vi "SampleSensorLoop.vi"   [LabVIEW 2016]
uses:
  DisplacementData.ctl
  DisplacementStates.ctl
  DisplacementSample.ctl
  DisplacementErrorSample.ctl
  DisplacementErrorCodes.ctl
  <vilib>/Platform/TimedLoop/XDataNode/timing_clust.ctl
  <vilib>/Platform/TimedLoop/XDataNode/nitl_modes.ctl
  <vilib>/Platform/TimedLoop/XDataNode/wakeup.ctl
  <vilib>/rvi/Emulation/niFpgaSctlEmulationGetInTimedLoop.vi
  <vilib>/rvi/Emulation/niFpgaEmulationReportErrorSimple.vi
  <vilib>/rvi/Emulation/niFpgaGetClockAttributes.vi
  <vilib>/rvi/Emulation/niFpgaCriticalErrorInLSC.vi
  <vilib>/rvi/Emulation/niFpgaEmulationIsFPGAContextNoSignature.vi
  <vilib>/rvi/errors/niFpgaSetErrorForExecOnDevCompSimple.vi
  <vilib>/rvi/eio/common/nirviEmuReportErrorAndStop.vi
  <vilib>/rvi/DataTransferAndStorage/Container/Common/niFpgaContainerGetUniqueNameForEmu.vi
  <vilib>/rvi/FIFO/Fifo_Resource/nirvififoEmulationSetSize.vi
  <vilib>/rvi/FIFO/Fifo_Resource/nirviFifoEmulationQueueMgr.vi
  <instcachedir>/0/nirviFifoEmulationQueueMgr_E5CAEC123FF24DC58D834DCA3CDAA9B5.lvgen/nirviFifoEmulationQueueMgr_E5CAEC123FF24DC58D834DCA3CDAA9B5_004.vi
  <vilib>/Utility/error.llb/Clear Errors.vi
  <vilib>/rvi/FIFO/Fifo_Resource/nirvififoEmulationCreateLock.vi
  <vilib>/rvi/Emulation/niFpgaProcessEmulError.vi
  <vilib>/rvi/FIFO/Fifo_Resource/nirvififoEmulationObtainLock.vi
  <vilib>/rvi/FIFO/Fifo_Resource/nirvififoEmulationReleaseLock.vi
  <vilib>/rvi/occurrence/nirviWaitOnOccurrenceBase.vi
  <vilib>/rvi/errors/nirviReportUnexpectedCaseInternalError.vi
  <vilib>/rvi/errors/nirviReportUnexpectedCaseInternalError (U32).vi
  <vilib>/rvi/FIFO/Fifo_Resource/nirvififoEmulationDetermineInputValidOut.vi
  <instcachedir>/0/nirviFifoEmulationQueueMgr_E5CAEC123FF24DC58D834DCA3CDAA9B5.lvgen/nirviFifoEmulationQueueMgr_E5CAEC123FF24DC58D834DCA3CDAA9B5_009.vi
  <vilib>/rvi/Memory/Memory_Emulation/niFpgaMemoryEmulationCacheClearOnFirstRun.vi
  <vilib>/rvi/Memory/Memory_Emulation/nirvimemoryEmulationManagerCache_MakeExclusive.vi
  <vilib>/rvi/Memory/Memory_Emulation/niFpgaMemoryEmulationValidateCache.vi
  <vilib>/rvi/Memory/Memory_Emulation/nirvimemoryEmulationManagerCache_InsertValue.vi
  <vilib>/rvi/Memory/Memory_Emulation/nirvimemoryEmulationManagerCache_ReleaseExclusive.vi
  <vilib>/rvi/Memory/Memory_Emulation/nirvimemoryEmulationManagerCache_GetValue.vi
  <vilib>/rvi/Memory/Memory_Emulation/nirvimemoryEmulationManagerCache_SetValue.vi
  <vilib>/rvi/eio/common/nirviEmuTemplateMethod_errors.vi
  <instcachedir>/0/nirviFifoEmulationQueueMgr_E5CAEC123FF24DC58D834DCA3CDAA9B5.lvgen/nirviFifoEmulationQueueMgr_E5CAEC123FF24DC58D834DCA3CDAA9B5_028.vi
  <instcachedir>/0/nirviFifoEmulationQueueMgr_E5CAEC123FF24DC58D834DCA3CDAA9B5.lvgen/nirviFifoEmulationQueueMgr_E5CAEC123FF24DC58D834DCA3CDAA9B5_029.vi
  <vilib>/Platform/TimedLoop/XDataNode/XDataNode.xnode
  <vilib>/rvi/DataTransferAndStorage/Container/XNode/niFpgaContainer.xnode
  <vilib>/rvi/FIFO/Fifo_Resource/nirvififoEmulationRead.vi
  <vilib>/rvi/FIFO/Fifo_Resource/nirvififoEmulationWrite.vi
  <vilib>/rvi/DataTransferAndStorage/Register/Emulation/niFpgaRegisterEmulation.vi
  <vilib>/eio/EIONode/EIONode.xnode
  <vilib>/Platform/TimedLoop/XDataNode/XDNodeRunTimeDep.lvlib
types:
  T1 = typedef "DisplacementData.ctl" = cluster{"State":T2, "Sensor":u8, "Negative":bool, "Timestamp":u64, "ErrorNumber":u8, "Timeout":i32, "Sample":T3, "ErrorSample":T4}
  T2 = typedef "DisplacementStates.ctl" = enum16{"WaitForTrigger", "ClearRxFIFO", "WaitForClearComplete", "WriteM", "Write0", "WriteCR", "WriteNL", "ReadFirstCharacter", "ReadDataResponse", "ReadDeliminator", "ReadSign", "ReadHundreds", "ReadTens", "ReadOnes", "ReadDecimal", "ReadTenths", "ReadHundredths", "ReadThousandths", "ReadTenThousandths", "PrepareSample", "MoveSample", "ReadErrorR", "ReadErrorDeliminator1", "ReadErrorM", "ReadError0", "ReadErrorDeliminator2", "ReadErrorNumberTens", "ReadErrorNumberOnes", "ReadErrorCR", "ParseErrorNumber", "ResponseUnknownError", "ResponseInvalidError", "ResponseTimeoutError", "SensorIndicatesInvalidCommandError", "SensorIndicatesCommunicationTimeoutError", "SensorIndicatesDataLengthError", "SensorIndicatesNumberOfParametersError", "SensorIndicatesParameterError", "SensorIndicatesCommunicationError", "SensorIndicatesIDNumberError", "SensorIndicatesExpansionLineError", "SensorIndicatesWriteControlError", "PrepareErrorCode", "MoveErrorCode"}
  T3 = typedef "DisplacementSample.ctl" = cluster{"Timestamp":u64, "TxBytes":u64, "RxBytes":u64, "TxFrames":u64, "RxFrames":u64, "Sensor1Raw":i32, "Sensor2Raw":i32, "Sensor3Raw":i32, "Sensor4Raw":i32, "Sensor5Raw":i32, "Sensor6Raw":i32, "Sensor7Raw":i32, "Sensor8Raw":i32, "Sensor1Eng":sgl, "Sensor2Eng":sgl, "Sensor3Eng":sgl, "Sensor4Eng":sgl, "Sensor5Eng":sgl, "Sensor6Eng":sgl, "Sensor7Eng":sgl, "Sensor8Eng":sgl, "PositionX":sgl, "PositionY":sgl, "PositionZ":sgl, "RotationX":sgl, "RotationY":sgl, "RotationZ":sgl}
  T4 = typedef "DisplacementErrorSample.ctl" = cluster{"Timestamp":u64, "TxBytes":u64, "RxBytes":u64, "TxFrames":u64, "RxFrames":u64, "ErrorCode":T5}
  T5 = typedef "DisplacementErrorCodes.ctl" = enum16{"None", "ResponseUnknownError", "ResponseInvalidError", "ResponseTimeoutError", "SensorIndicatesInvalidCommandError", "SensorIndicatesCommunicationTimeoutError", "SensorIndicatesDataLengthError", "SensorIndicatesNumberOfParametersError", "SensorIndicatesParameterError", "SensorIndicatesCommunicationError", "SensorIndicatesIDNumberError", "SensorIndicatesExpansionLineError", "SensorIndicatesWriteControlError"}
  T6 = typedef "XDNodeRunTimeDep.lvlib/timing_clust.ctl" = cluster{"Expected End [f-1]":u64, "Actual End [f-1]":u64, "Finished Late? [f-1]":bool, "Expected End [i-1]":u64, "Actual End [i-1]":u64, "Finished Late? [i-1]":bool, "Expected Start [i]":u64, "Actual Start [i]":u64, "Expected Start [f]":u64, "Actual Start [f]":u64, "Source Name":string, "Structure Name":string, "Period":i64, "Deadline":i64, "Offset":i64, "Start":i64, "Priority":i32, "Timeout":i32, "Mode":T7, "Wakeup Reason":T8, "Error":errorcluster, "Source Type":string, "Secondary Source Type":string, "Global End Time":u64, "Global Start Time":u64, "Frame Duration":u64, "Iteration Duration":u64, "Assigned CPU":i32, "I/O Scan Engine Mode":u32}
  T7 = typedef "XDNodeRunTimeDep.lvlib/nitl_modes.ctl" = enum32{"No Change", "Process missed periods, maintain original phase", "Discard missed periods, maintain original phase", "Process missed periods, ignore original phase", "Discard missed periods, ignore original phase"}
  T8 = typedef "XDNodeRunTimeDep.lvlib/wakeup.ctl" = enum32{"Normal", "Aborted", "Asynchronous wakeup", "Timing source error", "Timed loop error", "Timeout"}
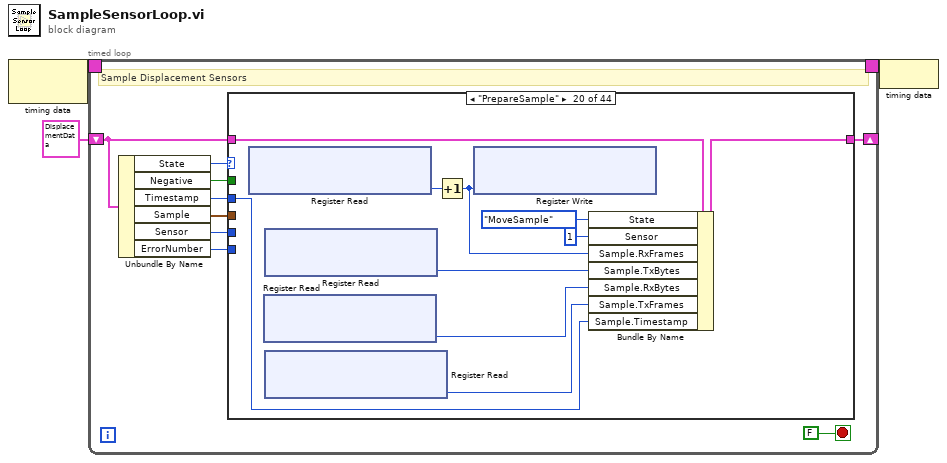
[diagram p0: block diagram]
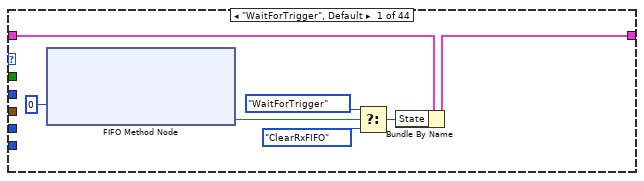
[diagram p2: hidden frame]
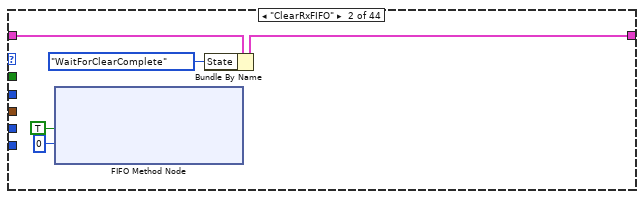
[diagram p3: hidden frame]
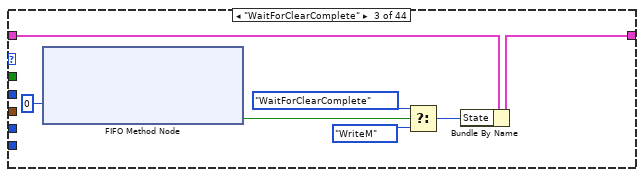
[diagram p4: hidden frame]
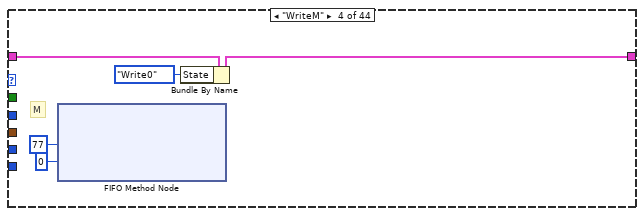
[diagram p5: hidden frame]
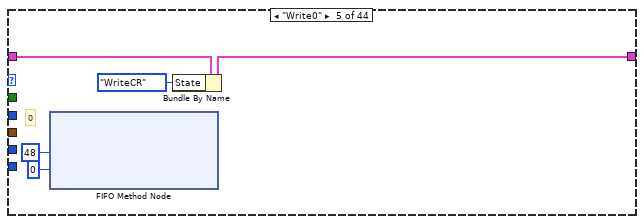
[diagram p6: hidden frame]
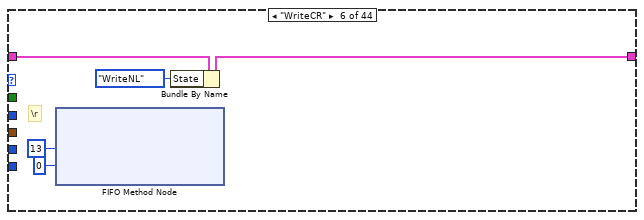
[diagram p7: hidden frame]
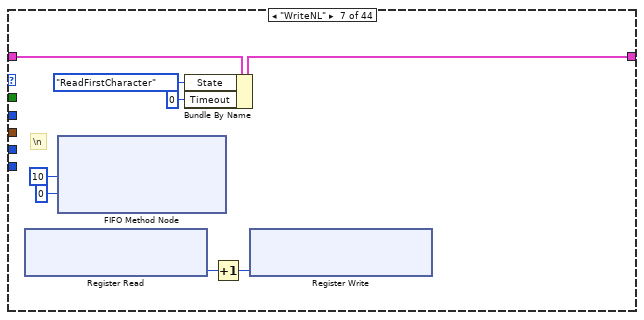
[diagram p8: hidden frame]
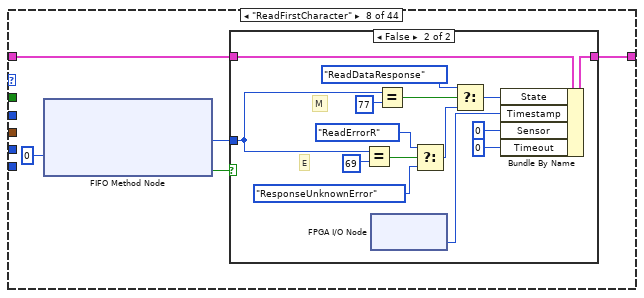
[diagram p9: hidden frame]
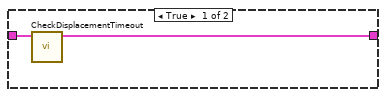
[diagram p10: hidden frame]
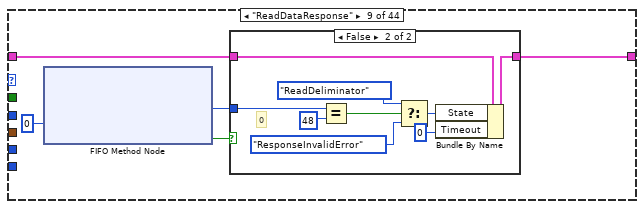
[diagram p11: hidden frame]
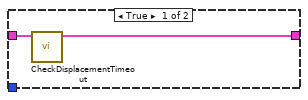
[diagram p12: hidden frame]
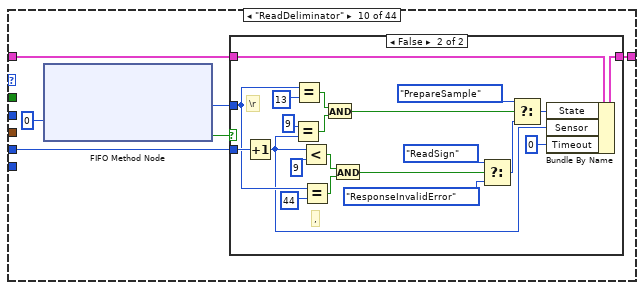
[diagram p13: hidden frame]
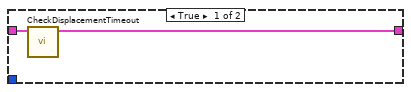
[diagram p14: hidden frame]
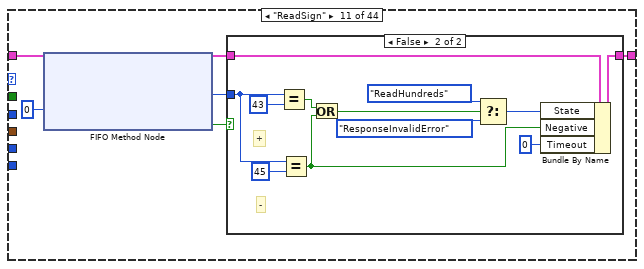
[diagram p15: hidden frame]
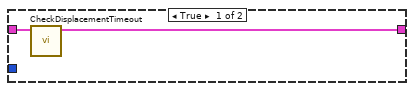
[diagram p16: hidden frame]
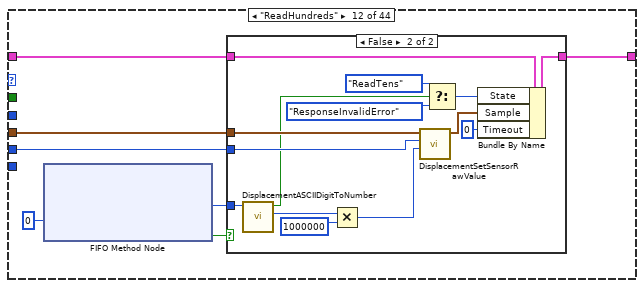
[diagram p17: hidden frame]
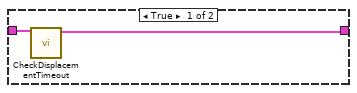
[diagram p18: hidden frame]
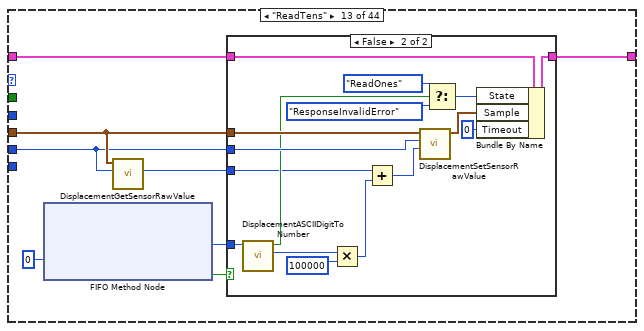
[diagram p19: hidden frame]
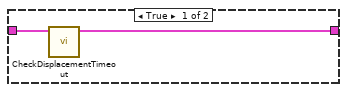
[diagram p20: hidden frame]
diagram:
  n1 = node-c288() -> (w3:T6)  [unwired: 1 in]
  n2 = timed-loop {
    timing: w3 -> [_]
    timing-out: [_] -> w2
    shift-right: [w12] -> _
    shift-left: T1 {"State"=enum."WaitForTrigger", "Sensor"=0, "Negative"=FALSE, "Timestamp"=0, "ErrorNumber"=0, "Timeout"=0, "Sample"={"Timestamp"=0, "TxBytes"=0, "RxBytes"=0, "TxFrames"=0, "RxFrames"=0, "Sensor1Raw"=0, "Sensor2Raw"=0, "Sensor3Raw"=0, "Sensor4Raw"=0, "Sensor5Raw"=0, "Sensor6Raw"=0, "Sensor7Raw"=0, "Sensor8Raw"=0, "Sensor1Eng"=0.0, "Sensor2Eng"=0.0, "Sensor3Eng"=0.0, "Sensor4Eng"=0.0, "Sensor5Eng"=0.0, "Sensor6Eng"=0.0, "Sensor7Eng"=0.0, "Sensor8Eng"=0.0, "PositionX"=0.0, "PositionY"=0.0, "PositionZ"=0.0, "RotationX"=0.0, "RotationY"=0.0, "RotationZ"=0.0}, "ErrorSample"={"Timestamp"=0, "TxBytes"=0, "RxBytes"=0, "TxFrames"=0, "RxFrames"=0, "ErrorCode"=enum."None"}} ("DisplacementData") -> [w11]
    stop <- FALSE stop-if-true
    # "Sample Displacement Sensors"
    n3 = Unbundle By Name(w11) -> ("State"=w10:T2, "Negative"=w9:bool, "Timestamp"=w7:u64, "Sample"=w8:T3, "Sensor"=w6:u8, "ErrorNumber"=w5:u8)
    n4 = case shown="\"PrepareSample\"" w10 {
      tunnel: [w16 w23 w30 w35 w40 w45 w53 w58 w80 w97 w125 w146 w170 w196 w219 w238 w264 w290 w316 w342 w349 w353 w369 w385 w401 w417 w433 w453 w472 w487 w501 w505 w509 w513 w517 w521 w525 w529 w533 w537 w541 w545 w555 w562] -> w12
      tunnel: w11 -> [w19 w24 w31 w36 w41 w46 w54 w59 w81 w98 w126 w147 w171 w197 w220 w239 w265 w291 w317 w343 w346 w354 w370 w386 w402 w418 w434 w454 w473 w488 w502 w506 w510 w514 w518 w522 w526 w530 w534 w538 w542 w546 w556 w559]
      tunnel: w9 -> [_ _ _ _ _ _ _ _ _ _ _ _ _ _ _ _ _ _ _ _ _ _ _ _ _ _ _ _ _ _ _ _ _ _ _ _ _ _ _ _ _ _ _ _]
      tunnel: w8 -> [_ _ _ _ _ _ _ _ _ _ _ w142 w166 w192 _ w234 w260 w286 w312 _ _ _ _ _ _ _ _ _ _ _ _ _ _ _ _ _ _ _ _ _ _ _ _ _]
      tunnel: w7 -> [_ _ _ _ _ _ _ _ _ _ _ _ _ _ _ _ _ _ _ w334 _ _ _ _ _ _ _ _ _ _ _ _ _ _ _ _ _ _ _ _ _ _ w547 _]
      tunnel: w6 -> [_ _ _ _ _ _ _ _ _ w93 _ w141 w165 w191 _ w233 w259 w285 w311 _ _ _ _ _ _ _ _ _ _ _ _ _ _ _ _ _ _ _ _ _ _ _ _ _]
      tunnel: w5 -> [_ _ _ _ _ _ _ _ _ _ _ _ _ _ _ _ _ _ _ _ _ _ _ _ _ _ _ w449 _ w485 _ _ _ _ _ _ _ _ _ _ _ _ _ _]
      frame "WaitForTrigger", Default {
        n5 = xnode ("FIFO Method Node")("Timeout"=0) -> ("Timed Out?"=w14:bool)  [unwired: 1 in, 2 out]
        n6 = Select(t=DisplacementStates."WaitForTrigger" ("DisplacementStates"), s=w14, f=DisplacementStates."ClearRxFIFO") -> (s? t:f=w17:T2)
        n7 = Bundle By Name(cluster=w19, "State"=w17) -> (w16:T1)
      }
      frame "ClearRxFIFO" {
        n8 = xnode ("FIFO Method Node")("Element"=TRUE, "Timeout"=0) -> ()  [unwired: 1 in, 2 out]
        n9 = Bundle By Name(cluster=w24, "State"=DisplacementStates."WaitForClearComplete") -> (w23:T1)
      }
      frame "WaitForClearComplete" {
        n10 = xnode ("FIFO Method Node")("Timeout"=0) -> ("Timed Out?"=w26:bool)  [unwired: 1 in, 2 out]
        n11 = Select(t=DisplacementStates."WaitForClearComplete" ("State"), s=w26, f=DisplacementStates."WriteM") -> (s? t:f=w28:T2)
        n12 = Bundle By Name(cluster=w31, "State"=w28) -> (w30:T1)
      }
      frame "WriteM" {
        # "M"
        n13 = xnode ("FIFO Method Node")("Element"=u8 77, "Timeout"=0) -> ()  [unwired: 1 in, 2 out]
        n14 = Bundle By Name(cluster=w36, "State"=DisplacementStates."Write0" ("f")) -> (w35:T1)
      }
      frame "Write0" {
        # "0"
        n15 = xnode ("FIFO Method Node")("Element"=u8 48, "Timeout"=0) -> ()  [unwired: 1 in, 2 out]
        n16 = Bundle By Name(cluster=w41, "State"=DisplacementStates."WriteCR" ("f")) -> (w40:T1)
      }
      frame "WriteCR" {
        # "\\r"
        n17 = xnode ("FIFO Method Node")("Element"=u8 13, "Timeout"=0) -> ()  [unwired: 1 in, 2 out]
        n18 = Bundle By Name(cluster=w46, "State"=DisplacementStates."WriteNL" ("f")) -> (w45:T1)
      }
      frame "WriteNL" {
        # "\\n"
        n19 = xnode ("Register Read")() -> ("Data"=w48:u64)  [unwired: 1 in, 1 out]
        n20 = xnode ("FIFO Method Node")("Element"=u8 10, "Timeout"=0) -> ()  [unwired: 1 in, 2 out]
        n21 = Bundle By Name(cluster=w54, "State"=DisplacementStates."ReadFirstCharacter", "Timeout"=0) -> (w53:T1)
        n22 = Increment(x=w48) -> (x+1=w49:u64)
        n23 = xnode ("Register Write")("Data"=w49) -> ()  [unwired: 1 in, 1 out]
      }
      frame "ReadFirstCharacter" {
        n24 = xnode ("FIFO Method Node")("Timeout"=0) -> ("Element"=w55:u8, "Timed Out?"=w56:bool)  [unwired: 1 in, 1 out]
        n25 = case shown="False" w56 {
          tunnel: w59 -> [w61 w76]
          tunnel: [w60 w75] -> w58
          tunnel: w55 -> [_ w68]
          frame True {
            n26 = call "CheckDisplacementTimeout.vi"("DisplacementData in"=w61) -> ("DisplacementData out"=w60:T1)  [unwired: 10 in]
          }
          frame False {
            # "E"
            # "M"
            n27 = Equal?(x=w68, y=u8 69) -> (x = y?=w69:bool)
            n28 = xnode "FPGA I/O Node"() -> ("Time"=w64:u64)  [unwired: 1 in, 1 out]
            n29 = Equal?(x=w68, y=u8 77) -> (x = y?=w73:bool)
            n30 = Select(t=DisplacementStates."ReadErrorR", s=w69, f=DisplacementStates."ResponseUnknownError") -> (s? t:f=w66:T2)
            n31 = Select(t=DisplacementStates."ReadDataResponse" ("State"), s=w73, f=w66) -> (s? t:f=w72:T2)
            n32 = Bundle By Name(cluster=w76, "State"=w72, "Timestamp"=w64, "Sensor"=u8 0, "Timeout"=0) -> (w75:T1)
          }
        }
      }
      frame "ReadDataResponse" {
        n33 = xnode ("FIFO Method Node")("Timeout"=0) -> ("Element"=w77:u8, "Timed Out?"=w78:bool)  [unwired: 1 in, 1 out]
        n34 = case shown="False" w78 {
          tunnel: w81 -> [w83 w92]
          tunnel: [w82 w91] -> w80
          tunnel: w77 -> [_ w86]
          frame True {
            n35 = call "CheckDisplacementTimeout.vi"("DisplacementData in"=w83) -> ("DisplacementData out"=w82:T1)  [unwired: 10 in]
          }
          frame False {
            # "0"
            n36 = Equal?(x=w86, y=u8 48) -> (x = y?=w89:bool)
            n37 = Select(t=DisplacementStates."ReadDeliminator" ("State"), s=w89, f=DisplacementStates."ResponseInvalidError") -> (s? t:f=w88:T2)
            n38 = Bundle By Name(cluster=w92, "State"=w88, "Timeout"=0) -> (w91:T1)
          }
        }
      }
      frame "ReadDeliminator" {
        n39 = xnode ("FIFO Method Node")("Timeout"=0) -> ("Element"=w94:u8, "Timed Out?"=w95:bool)  [unwired: 1 in, 1 out]
        n40 = case shown="False" w95 {
          tunnel: w98 -> [w100 w121]
          tunnel: [w99 w120] -> w97
          tunnel: w94 -> [_ w110]
          tunnel: w93 -> [_ w117]
          frame True {
            n41 = call "CheckDisplacementTimeout.vi"("DisplacementData in"=w100) -> ("DisplacementData out"=w99:T1)  [unwired: 10 in]
          }
          frame False {
            # "\\r"
            # ","
            n42 = Increment(x=w117) -> (x+1=w102:u8)
            n43 = Equal?(x=u8 9, y=w102) -> (x = y?=w109:bool)
            n44 = Equal?(x=w110, y=u8 13) -> (x = y?=w108:bool)
            n45 = Less?(x=w102, y=u8 9) -> (x < y?=w115:bool)
            n46 = Equal?(x=w110, y=u8 44) -> (x = y?=w114:bool)
            n47 = And(x=w108, y=w109) -> (x .and. y?=w106:bool)
            n48 = And(x=w115, y=w114) -> (x .and. y?=w103:bool)
            n49 = Select(t=DisplacementStates."ReadSign" ("State"), s=w103, f=DisplacementStates."ResponseInvalidError") -> (s? t:f=w107:T2)
            n50 = Select(t=DisplacementStates."PrepareSample", s=w106, f=w107) -> (s? t:f=w104:T2)
            n51 = Bundle By Name(cluster=w121, "State"=w104, "Sensor"=w102, "Timeout"=0) -> (w120:T1)
          }
        }
      }
      frame "ReadSign" {
        n52 = xnode ("FIFO Method Node")("Timeout"=0) -> ("Element"=w122:u8, "Timed Out?"=w123:bool)  [unwired: 1 in, 1 out]
        n53 = case shown="False" w123 {
          tunnel: w126 -> [w128 w140]
          tunnel: [w127 w139] -> w125
          tunnel: w122 -> [_ w136]
          frame True {
            n54 = call "CheckDisplacementTimeout.vi"("DisplacementData in"=w128) -> ("DisplacementData out"=w127:T1)  [unwired: 10 in]
          }
          frame False {
            # "+"
            # "-"
            n55 = Equal?(x=w136, y=u8 43) -> (x = y?=w137:bool)
            n56 = Equal?(x=w136, y=u8 45) -> (x = y?=w134:bool)
            n57 = Or(x=w137, y=w134) -> (x .or. y?=w133:bool)
            n58 = Select(t=DisplacementStates."ReadHundreds" ("State"), s=w133, f=DisplacementStates."ResponseInvalidError") -> (s? t:f=w131:T2)
            n59 = Bundle By Name(cluster=w140, "State"=w131, "Negative"=w134, "Timeout"=0) -> (w139:T1)
          }
        }
      }
      frame "ReadHundreds" {
        n60 = xnode ("FIFO Method Node")("Timeout"=0) -> ("Element"=w143:u8, "Timed Out?"=w144:bool)  [unwired: 1 in, 1 out]
        n61 = case shown="False" w144 {
          tunnel: w147 -> [w149 w163]
          tunnel: [w148 w162] -> w146
          tunnel: w143 -> [_ w153]
          tunnel: w142 -> [_ w156]
          tunnel: w141 -> [_ w154]
          frame True {
            n62 = call "CheckDisplacementTimeout.vi"("DisplacementData in"=w149) -> ("DisplacementData out"=w148:T1)  [unwired: 10 in]
          }
          frame False {
            n63 = call "DisplacementASCIIDigitToNumber.vi"("Value"=w153) -> ("Number"=w151:i32, "Valid"=w152:bool)  [unwired: 9 in]
            n64 = Multiply(x=w151, y=1000000) -> (x*y=w157:i32)
            n65 = call "DisplacementSetSensorRawValue.vi"("Value"=w157, "Sensor"=w154, "DisplacementSample in"=w156) -> ("DisplacementSample out"=w155:T3)  [unwired: 8 in]
            n66 = Select(t=DisplacementStates."ReadTens" ("State"), s=w152, f=DisplacementStates."ResponseInvalidError" ("State")) -> (s? t:f=w160:T2)
            n67 = Bundle By Name(cluster=w163, "State"=w160, "Sample"=w155, "Timeout"=0) -> (w162:T1)
          }
        }
      }
      frame "ReadTens" {
        n68 = xnode ("FIFO Method Node")("Timeout"=0) -> ("Element"=w167:u8, "Timed Out?"=w168:bool)  [unwired: 1 in, 1 out]
        n69 = call "DisplacementGetSensorRawValue.vi"("Sensor"=w165, "DisplacementSample"=w166) -> ("Value"=w164:i32)  [unwired: 9 in]
        n70 = case shown="False" w168 {
          tunnel: w171 -> [w173 w189]
          tunnel: [w172 w188] -> w170
          tunnel: w167 -> [_ w180]
          tunnel: w166 -> [_ w183]
          tunnel: w165 -> [_ w181]
          tunnel: w164 -> [_ w177]
          frame True {
            n71 = call "CheckDisplacementTimeout.vi"("DisplacementData in"=w173) -> ("DisplacementData out"=w172:T1)  [unwired: 10 in]
          }
          frame False {
            n72 = call "DisplacementASCIIDigitToNumber.vi"("Value"=w180) -> ("Number"=w178:i32, "Valid"=w179:bool)  [unwired: 9 in]
            n73 = Multiply(x=w178, y=100000) -> (x*y=w175:i32)
            n74 = Add(x=w177, y=w175) -> (x+y=w176:i32)
            n75 = call "DisplacementSetSensorRawValue.vi"("Value"=w176, "Sensor"=w181, "DisplacementSample in"=w183) -> ("DisplacementSample out"=w182:T3)  [unwired: 8 in]
            n76 = Select(t=DisplacementStates."ReadOnes" ("State"), s=w179, f=DisplacementStates."ResponseInvalidError" ("State")) -> (s? t:f=w186:T2)
            n77 = Bundle By Name(cluster=w189, "State"=w186, "Sample"=w182, "Timeout"=0) -> (w188:T1)
          }
        }
      }
      frame "ReadOnes" {
        n78 = xnode ("FIFO Method Node")("Timeout"=0) -> ("Element"=w193:u8, "Timed Out?"=w194:bool)  [unwired: 1 in, 1 out]
        n79 = call "DisplacementGetSensorRawValue.vi"("Sensor"=w191, "DisplacementSample"=w192) -> ("Value"=w190:i32)  [unwired: 9 in]
        n80 = case shown="False" w194 {
          tunnel: w197 -> [w199 w215]
          tunnel: [w198 w214] -> w196
          tunnel: w193 -> [_ w206]
          tunnel: w192 -> [_ w209]
          tunnel: w191 -> [_ w207]
          tunnel: w190 -> [_ w203]
          frame True {
            n81 = call "CheckDisplacementTimeout.vi"("DisplacementData in"=w199) -> ("DisplacementData out"=w198:T1)  [unwired: 10 in]
          }
          frame False {
            n82 = call "DisplacementASCIIDigitToNumber.vi"("Value"=w206) -> ("Number"=w204:i32, "Valid"=w205:bool)  [unwired: 9 in]
            n83 = Multiply(x=w204, y=10000) -> (x*y=w201:i32)
            n84 = Add(x=w203, y=w201) -> (x+y=w202:i32)
            n85 = call "DisplacementSetSensorRawValue.vi"("Value"=w202, "Sensor"=w207, "DisplacementSample in"=w209) -> ("DisplacementSample out"=w208:T3)  [unwired: 8 in]
            n86 = Select(t=DisplacementStates."ReadDecimal" ("State"), s=w205, f=DisplacementStates."ResponseInvalidError" ("State")) -> (s? t:f=w212:T2)
            n87 = Bundle By Name(cluster=w215, "State"=w212, "Sample"=w208, "Timeout"=0) -> (w214:T1)
          }
        }
      }
      frame "ReadDecimal" {
        n88 = xnode ("FIFO Method Node")("Timeout"=0) -> ("Element"=w216:u8, "Timed Out?"=w217:bool)  [unwired: 1 in, 1 out]
        n89 = case shown="False" w217 {
          tunnel: w220 -> [w222 w231]
          tunnel: [w221 w230] -> w219
          tunnel: w216 -> [_ w226]
          frame True {
            n90 = call "CheckDisplacementTimeout.vi"("DisplacementData in"=w222) -> ("DisplacementData out"=w221:T1)  [unwired: 10 in]
          }
          frame False {
            # "."
            n91 = Equal?(x=w226, y=u8 46) -> (x = y?=w224:bool)
            n92 = Select(t=DisplacementStates."ReadTenths" ("State"), s=w224, f=DisplacementStates."ResponseInvalidError" ("State")) -> (s? t:f=w229:T2)
            n93 = Bundle By Name(cluster=w231, "State"=w229, "Timeout"=0) -> (w230:T1)
          }
        }
      }
      frame "ReadTenths" {
        n94 = xnode ("FIFO Method Node")("Timeout"=0) -> ("Element"=w235:u8, "Timed Out?"=w236:bool)  [unwired: 1 in, 1 out]
        n95 = call "DisplacementGetSensorRawValue.vi"("Sensor"=w233, "DisplacementSample"=w234) -> ("Value"=w232:i32)  [unwired: 9 in]
        n96 = case shown="False" w236 {
          tunnel: w239 -> [w241 w257]
          tunnel: [w240 w256] -> w238
          tunnel: w235 -> [_ w248]
          tunnel: w234 -> [_ w251]
          tunnel: w233 -> [_ w249]
          tunnel: w232 -> [_ w245]
          frame True {
            n97 = call "CheckDisplacementTimeout.vi"("DisplacementData in"=w241) -> ("DisplacementData out"=w240:T1)  [unwired: 10 in]
          }
          frame False {
            n98 = call "DisplacementASCIIDigitToNumber.vi"("Value"=w248) -> ("Number"=w246:i32, "Valid"=w247:bool)  [unwired: 9 in]
            n99 = Multiply(x=w246, y=1000) -> (x*y=w243:i32)
            n100 = Add(x=w245, y=w243) -> (x+y=w244:i32)
            n101 = call "DisplacementSetSensorRawValue.vi"("Value"=w244, "Sensor"=w249, "DisplacementSample in"=w251) -> ("DisplacementSample out"=w250:T3)  [unwired: 8 in]
            n102 = Select(t=DisplacementStates."ReadHundredths" ("State"), s=w247, f=DisplacementStates."ResponseInvalidError" ("State")) -> (s? t:f=w254:T2)
            n103 = Bundle By Name(cluster=w257, "State"=w254, "Sample"=w250, "Timeout"=0) -> (w256:T1)
          }
        }
      }
      frame "ReadHundredths" {
        n104 = xnode ("FIFO Method Node")("Timeout"=0) -> ("Element"=w261:u8, "Timed Out?"=w262:bool)  [unwired: 1 in, 1 out]
        n105 = call "DisplacementGetSensorRawValue.vi"("Sensor"=w259, "DisplacementSample"=w260) -> ("Value"=w258:i32)  [unwired: 9 in]
        n106 = case shown="False" w262 {
          tunnel: w265 -> [w267 w283]
          tunnel: [w266 w282] -> w264
          tunnel: w261 -> [_ w274]
          tunnel: w260 -> [_ w277]
          tunnel: w259 -> [_ w275]
          tunnel: w258 -> [_ w271]
          frame True {
            n107 = call "CheckDisplacementTimeout.vi"("DisplacementData in"=w267) -> ("DisplacementData out"=w266:T1)  [unwired: 10 in]
          }
          frame False {
            n108 = call "DisplacementASCIIDigitToNumber.vi"("Value"=w274) -> ("Number"=w272:i32, "Valid"=w273:bool)  [unwired: 9 in]
            n109 = Multiply(x=w272, y=100) -> (x*y=w269:i32)
            n110 = Add(x=w271, y=w269) -> (x+y=w270:i32)
            n111 = call "DisplacementSetSensorRawValue.vi"("Value"=w270, "Sensor"=w275, "DisplacementSample in"=w277) -> ("DisplacementSample out"=w276:T3)  [unwired: 8 in]
            n112 = Select(t=DisplacementStates."ReadThousandths" ("State"), s=w273, f=DisplacementStates."ResponseInvalidError" ("State")) -> (s? t:f=w280:T2)
            n113 = Bundle By Name(cluster=w283, "State"=w280, "Sample"=w276, "Timeout"=0) -> (w282:T1)
          }
        }
      }
      frame "ReadThousandths" {
        n114 = xnode ("FIFO Method Node")("Timeout"=0) -> ("Element"=w287:u8, "Timed Out?"=w288:bool)  [unwired: 1 in, 1 out]
        n115 = call "DisplacementGetSensorRawValue.vi"("Sensor"=w285, "DisplacementSample"=w286) -> ("Value"=w284:i32)  [unwired: 9 in]
        n116 = case shown="False" w288 {
          tunnel: w291 -> [w293 w309]
          tunnel: [w292 w308] -> w290
          tunnel: w287 -> [_ w300]
          tunnel: w286 -> [_ w303]
          tunnel: w285 -> [_ w301]
          tunnel: w284 -> [_ w297]
          frame True {
            n117 = call "CheckDisplacementTimeout.vi"("DisplacementData in"=w293) -> ("DisplacementData out"=w292:T1)  [unwired: 10 in]
          }
          frame False {
            n118 = call "DisplacementASCIIDigitToNumber.vi"("Value"=w300) -> ("Number"=w298:i32, "Valid"=w299:bool)  [unwired: 9 in]
            n119 = Multiply(x=w298, y=10) -> (x*y=w295:i32)
            n120 = Add(x=w297, y=w295) -> (x+y=w296:i32)
            n121 = call "DisplacementSetSensorRawValue.vi"("Value"=w296, "Sensor"=w301, "DisplacementSample in"=w303) -> ("DisplacementSample out"=w302:T3)  [unwired: 8 in]
            n122 = Select(t=DisplacementStates."ReadTenThousandths" ("State"), s=w299, f=DisplacementStates."ResponseInvalidError" ("State")) -> (s? t:f=w306:T2)
            n123 = Bundle By Name(cluster=w309, "State"=w306, "Sample"=w302, "Timeout"=0) -> (w308:T1)
          }
        }
      }
      frame "ReadTenThousandths" {
        n124 = xnode ("FIFO Method Node")("Timeout"=0) -> ("Element"=w313:u8, "Timed Out?"=w314:bool)  [unwired: 1 in, 1 out]
        n125 = call "DisplacementGetSensorRawValue.vi"("Sensor"=w311, "DisplacementSample"=w312) -> ("Value"=w310:i32)  [unwired: 9 in]
        n126 = case shown="False" w314 {
          tunnel: w317 -> [w319 w333]
          tunnel: [w318 w332] -> w316
          tunnel: w313 -> [_ w325]
          tunnel: w312 -> [_ w328]
          tunnel: w311 -> [_ w326]
          tunnel: w310 -> [_ w323]
          frame True {
            n127 = call "CheckDisplacementTimeout.vi"("DisplacementData in"=w319) -> ("DisplacementData out"=w318:T1)  [unwired: 10 in]
          }
          frame False {
            n128 = call "DisplacementASCIIDigitToNumber.vi"("Value"=w325) -> ("Number"=w321:i32, "Valid"=w324:bool)  [unwired: 9 in]
            n129 = Add(x=w323, y=w321) -> (x+y=w322:i32)
            n130 = call "DisplacementSetSensorRawValue.vi"("Value"=w322, "Sensor"=w326, "DisplacementSample in"=w328) -> ("DisplacementSample out"=w327:T3)  [unwired: 8 in]
            n131 = Select(t=DisplacementStates."ReadDeliminator" ("State"), s=w324, f=DisplacementStates."ResponseInvalidError" ("State")) -> (s? t:f=w331:T2)
            n132 = Bundle By Name(cluster=w333, "State"=w331, "Sample"=w327, "Timeout"=0) -> (w332:T1)
          }
        }
      }
      frame "PrepareSample" {
        n133 = xnode ("Register Read")() -> ("Data"=w340:u64)  [unwired: 1 in, 1 out]
        n134 = xnode ("Register Read")() -> ("Data"=w336:u64)  [unwired: 1 in, 1 out]
        n135 = xnode ("Register Read")() -> ("Data"=w337:u64)  [unwired: 1 in, 1 out]
        n136 = xnode ("Register Read")() -> ("Data"=w335:u64)  [unwired: 1 in, 1 out]
        n137 = Increment(x=w340) -> (x+1=w338:u64)
        n138 = xnode ("Register Write")("Data"=w338) -> ()  [unwired: 1 in, 1 out]
        n139 = Bundle By Name(cluster=w343, "State"=DisplacementStates."MoveSample", "Sensor"=u8 1, "Sample.RxFrames"=w338, "Sample.TxBytes"=w337, "Sample.RxBytes"=w336, "Sample.TxFrames"=w335, "Sample.Timestamp"=w334) -> (w342:T1)
      }
      frame "MoveSample" {
        n140 = Unbundle By Name(w346) -> ("Sample"=w344:T3)
        n141 = xnode ("FIFO Method Node")("Element"=w344, "Timeout"=0) -> ()  [unwired: 1 in, 2 out]
        n142 = Bundle By Name(cluster=w346, "State"=DisplacementStates."WaitForTrigger", "Sensor"=u8 1) -> (w349:T1)
      }
      frame "ReadErrorR" {
        n143 = xnode ("FIFO Method Node")("Timeout"=0) -> ("Element"=w350:u8, "Timed Out?"=w351:bool)  [unwired: 1 in, 1 out]
        n144 = case shown="False" w351 {
          tunnel: w354 -> [w356 w365]
          tunnel: [w355 w364] -> w353
          tunnel: w350 -> [_ w359]
          frame True {
            n145 = call "CheckDisplacementTimeout.vi"("DisplacementData in"=w356) -> ("DisplacementData out"=w355:T1)  [unwired: 10 in]
          }
          frame False {
            # "R"
            n146 = Equal?(x=w359, y=u8 82) -> (x = y?=w362:bool)
            n147 = Select(t=DisplacementStates."ReadErrorDeliminator1" ("State"), s=w362, f=DisplacementStates."ResponseInvalidError") -> (s? t:f=w361:T2)
            n148 = Bundle By Name(cluster=w365, "State"=w361, "Timeout"=0) -> (w364:T1)
          }
        }
      }
      frame "ReadErrorDeliminator1" {
        n149 = xnode ("FIFO Method Node")("Timeout"=0) -> ("Element"=w366:u8, "Timed Out?"=w367:bool)  [unwired: 1 in, 1 out]
        n150 = case shown="False" w367 {
          tunnel: w370 -> [w372 w381]
          tunnel: [w371 w380] -> w369
          tunnel: w366 -> [_ w376]
          frame True {
            n151 = call "CheckDisplacementTimeout.vi"("DisplacementData in"=w372) -> ("DisplacementData out"=w371:T1)  [unwired: 10 in]
          }
          frame False {
            # ","
            n152 = Equal?(x=w376, y=u8 44) -> (x = y?=w375:bool)
            n153 = Select(t=DisplacementStates."ReadErrorM" ("State"), s=w375, f=DisplacementStates."ResponseInvalidError") -> (s? t:f=w374:T2)
            n154 = Bundle By Name(cluster=w381, "State"=w374, "Timeout"=0) -> (w380:T1)
          }
        }
      }
      frame "ReadErrorM" {
        n155 = xnode ("FIFO Method Node")("Timeout"=0) -> ("Element"=w382:u8, "Timed Out?"=w383:bool)  [unwired: 1 in, 1 out]
        n156 = case shown="False" w383 {
          tunnel: w386 -> [w388 w397]
          tunnel: [w387 w396] -> w385
          tunnel: w382 -> [_ w391]
          frame True {
            n157 = call "CheckDisplacementTimeout.vi"("DisplacementData in"=w388) -> ("DisplacementData out"=w387:T1)  [unwired: 10 in]
          }
          frame False {
            # "M"
            n158 = Equal?(x=w391, y=u8 77) -> (x = y?=w394:bool)
            n159 = Select(t=DisplacementStates."ReadError0" ("State"), s=w394, f=DisplacementStates."ResponseInvalidError") -> (s? t:f=w393:T2)
            n160 = Bundle By Name(cluster=w397, "State"=w393, "Timeout"=0) -> (w396:T1)
          }
        }
      }
      frame "ReadError0" {
        n161 = xnode ("FIFO Method Node")("Timeout"=0) -> ("Element"=w398:u8, "Timed Out?"=w399:bool)  [unwired: 1 in, 1 out]
        n162 = case shown="False" w399 {
          tunnel: w402 -> [w404 w413]
          tunnel: [w403 w412] -> w401
          tunnel: w398 -> [_ w407]
          frame True {
            n163 = call "CheckDisplacementTimeout.vi"("DisplacementData in"=w404) -> ("DisplacementData out"=w403:T1)  [unwired: 10 in]
          }
          frame False {
            # "0"
            n164 = Equal?(x=w407, y=u8 48) -> (x = y?=w410:bool)
            n165 = Select(t=DisplacementStates."ReadErrorDeliminator2" ("State"), s=w410, f=DisplacementStates."ResponseInvalidError") -> (s? t:f=w409:T2)
            n166 = Bundle By Name(cluster=w413, "State"=w409, "Timeout"=0) -> (w412:T1)
          }
        }
      }
      frame "ReadErrorDeliminator2" {
        n167 = xnode ("FIFO Method Node")("Timeout"=0) -> ("Element"=w414:u8, "Timed Out?"=w415:bool)  [unwired: 1 in, 1 out]
        n168 = case shown="False" w415 {
          tunnel: w418 -> [w420 w429]
          tunnel: [w419 w428] -> w417
          tunnel: w414 -> [_ w424]
          frame True {
            n169 = call "CheckDisplacementTimeout.vi"("DisplacementData in"=w420) -> ("DisplacementData out"=w419:T1)  [unwired: 10 in]
          }
          frame False {
            # ","
            n170 = Equal?(x=w424, y=u8 44) -> (x = y?=w423:bool)
            n171 = Select(t=DisplacementStates."ReadErrorNumberTens" ("State"), s=w423, f=DisplacementStates."ResponseInvalidError") -> (s? t:f=w422:T2)
            n172 = Bundle By Name(cluster=w429, "State"=w422, "Timeout"=0) -> (w428:T1)
          }
        }
      }
      frame "ReadErrorNumberTens" {
        n173 = xnode ("FIFO Method Node")("Timeout"=0) -> ("Element"=w430:u8, "Timed Out?"=w431:bool)  [unwired: 1 in, 1 out]
        n174 = case shown="False" w431 {
          tunnel: w434 -> [w436 w448]
          tunnel: [w435 w447] -> w433
          tunnel: w430 -> [_ w441]
          frame True {
            n175 = call "CheckDisplacementTimeout.vi"("DisplacementData in"=w436) -> ("DisplacementData out"=w435:T1)  [unwired: 10 in]
          }
          frame False {
            n176 = call "DisplacementASCIIDigitToNumber.vi"("Value"=w441) -> ("Number"=w438:i32, "Valid"=w440:bool)  [unwired: 9 in]
            n177 = To Unsigned Byte Integer(number=w438) -> (unsigned 8bit integer=w439:u8)
            n178 = Multiply(x=w439, y=u8 10) -> (x*y=w442:u8)
            n179 = Select(t=DisplacementStates."ReadErrorNumberOnes" ("State"), s=w440, f=DisplacementStates."ResponseInvalidError" ("State")) -> (s? t:f=w445:T2)
            n180 = Bundle By Name(cluster=w448, "State"=w445, "ErrorNumber"=w442, "Timeout"=0) -> (w447:T1)
          }
        }
      }
      frame "ReadErrorNumberOnes" {
        n181 = xnode ("FIFO Method Node")("Timeout"=0) -> ("Element"=w450:u8, "Timed Out?"=w451:bool)  [unwired: 1 in, 1 out]
        n182 = case shown="False" w451 {
          tunnel: w454 -> [w456 w468]
          tunnel: [w455 w467] -> w453
          tunnel: w450 -> [_ w461]
          tunnel: w449 -> [_ w462]
          frame True {
            n183 = call "CheckDisplacementTimeout.vi"("DisplacementData in"=w456) -> ("DisplacementData out"=w455:T1)  [unwired: 10 in]
          }
          frame False {
            n184 = call "DisplacementASCIIDigitToNumber.vi"("Value"=w461) -> ("Number"=w459:i32, "Valid"=w460:bool)  [unwired: 9 in]
            n185 = To Unsigned Byte Integer(number=w459) -> (unsigned 8bit integer=w458:u8)
            n186 = Add(x=w462, y=w458) -> (x+y=w463:u8)
            n187 = Select(t=DisplacementStates."ReadErrorCR" ("State"), s=w460, f=DisplacementStates."ResponseInvalidError" ("State")) -> (s? t:f=w466:T2)
            n188 = Bundle By Name(cluster=w468, "State"=w466, "ErrorNumber"=w463, "Timeout"=0) -> (w467:T1)
          }
        }
      }
      frame "ReadErrorCR" {
        n189 = xnode ("FIFO Method Node")("Timeout"=0) -> ("Element"=w469:u8, "Timed Out?"=w470:bool)  [unwired: 1 in, 1 out]
        n190 = case shown="False" w470 {
          tunnel: w473 -> [w475 w484]
          tunnel: [w474 w483] -> w472
          tunnel: w469 -> [_ w479]
          frame True {
            n191 = call "CheckDisplacementTimeout.vi"("DisplacementData in"=w475) -> ("DisplacementData out"=w474:T1)  [unwired: 10 in]
          }
          frame False {
            # "\\r"
            n192 = Equal?(x=w479, y=u8 13) -> (x = y?=w478:bool)
            n193 = Select(t=DisplacementStates."ParseErrorNumber" ("State"), s=w478, f=DisplacementStates."ResponseInvalidError") -> (s? t:f=w477:T2)
            n194 = Bundle By Name(cluster=w484, "State"=w477, "Timeout"=0) -> (w483:T1)
          }
        }
      }
      frame "ParseErrorNumber" {
        n195 = case shown="255, Default" w485 {
          tunnel: [DisplacementStates."ResponseInvalidError" ("State") DisplacementStates."SensorIndicatesInvalidCommandError" ("State") DisplacementStates."SensorIndicatesCommunicationTimeoutError" ("State") DisplacementStates."SensorIndicatesDataLengthError" ("State") DisplacementStates."SensorIndicatesNumberOfParametersError" ("State") DisplacementStates."SensorIndicatesParameterError" ("State") DisplacementStates."SensorIndicatesCommunicationError" ("State") DisplacementStates."SensorIndicatesIDNumberError" ("State") DisplacementStates."SensorIndicatesExpansionLineError" ("State") DisplacementStates."SensorIndicatesWriteControlError" ("State")] -> w486
          frame 255, Default {
          }
          frame 0 {
          }
          frame 2 {
          }
          frame 20 {
          }
          frame 21 {
          }
          frame 22 {
          }
          frame 29 {
          }
          frame 65 {
          }
          frame 66 {
          }
          frame 67 {
          }
        }
        n196 = Bundle By Name(cluster=w488, "State"=w486) -> (w487:T1)
      }
      frame "ResponseUnknownError" {
        n197 = Bundle By Name(cluster=w502, "State"=DisplacementStates."PrepareErrorCode", "ErrorSample.ErrorCode"=DisplacementErrorCodes."ResponseUnknownError" ("DisplacementErrorCodes")) -> (w501:T1)
      }
      frame "ResponseInvalidError" {
        n198 = Bundle By Name(cluster=w506, "State"=DisplacementStates."PrepareErrorCode", "ErrorSample.ErrorCode"=DisplacementErrorCodes."ResponseInvalidError" ("DisplacementErrorCodes")) -> (w505:T1)
      }
      frame "ResponseTimeoutError" {
        n199 = Bundle By Name(cluster=w510, "State"=DisplacementStates."PrepareErrorCode", "ErrorSample.ErrorCode"=DisplacementErrorCodes."ResponseTimeoutError" ("DisplacementErrorCodes")) -> (w509:T1)
      }
      frame "SensorIndicatesInvalidCommandError" {
        n200 = Bundle By Name(cluster=w514, "State"=DisplacementStates."PrepareErrorCode", "ErrorSample.ErrorCode"=DisplacementErrorCodes."SensorIndicatesInvalidCommandError" ("DisplacementErrorCodes")) -> (w513:T1)
      }
      frame "SensorIndicatesCommunicationTimeoutError" {
        n201 = Bundle By Name(cluster=w518, "State"=DisplacementStates."PrepareErrorCode", "ErrorSample.ErrorCode"=DisplacementErrorCodes."SensorIndicatesCommunicationTimeoutError" ("DisplacementErrorCodes")) -> (w517:T1)
      }
      frame "SensorIndicatesDataLengthError" {
        n202 = Bundle By Name(cluster=w522, "State"=DisplacementStates."PrepareErrorCode", "ErrorSample.ErrorCode"=DisplacementErrorCodes."SensorIndicatesDataLengthError" ("DisplacementErrorCodes")) -> (w521:T1)
      }
      frame "SensorIndicatesNumberOfParametersError" {
        n203 = Bundle By Name(cluster=w526, "State"=DisplacementStates."PrepareErrorCode", "ErrorSample.ErrorCode"=DisplacementErrorCodes."SensorIndicatesNumberOfParametersError" ("DisplacementErrorCodes")) -> (w525:T1)
      }
      frame "SensorIndicatesParameterError" {
        n204 = Bundle By Name(cluster=w530, "State"=DisplacementStates."PrepareErrorCode", "ErrorSample.ErrorCode"=DisplacementErrorCodes."SensorIndicatesParameterError" ("DisplacementErrorCodes")) -> (w529:T1)
      }
      frame "SensorIndicatesCommunicationError" {
        n205 = Bundle By Name(cluster=w534, "State"=DisplacementStates."PrepareErrorCode", "ErrorSample.ErrorCode"=DisplacementErrorCodes."SensorIndicatesCommunicationError" ("DisplacementErrorCodes")) -> (w533:T1)
      }
      frame "SensorIndicatesIDNumberError" {
        n206 = Bundle By Name(cluster=w538, "State"=DisplacementStates."PrepareErrorCode", "ErrorSample.ErrorCode"=DisplacementErrorCodes."SensorIndicatesIDNumberError" ("DisplacementErrorCodes")) -> (w537:T1)
      }
      frame "SensorIndicatesExpansionLineError" {
        n207 = Bundle By Name(cluster=w542, "State"=DisplacementStates."PrepareErrorCode", "ErrorSample.ErrorCode"=DisplacementErrorCodes."SensorIndicatesExpansionLineError" ("DisplacementErrorCodes")) -> (w541:T1)
      }
      frame "SensorIndicatesWriteControlError" {
        n208 = Bundle By Name(cluster=w546, "State"=DisplacementStates."PrepareErrorCode", "ErrorSample.ErrorCode"=DisplacementErrorCodes."SensorIndicatesWriteControlError" ("DisplacementErrorCodes")) -> (w545:T1)
      }
      frame "PrepareErrorCode" {
        n209 = xnode ("Register Read")() -> ("Data"=w553:u64)  [unwired: 1 in, 1 out]
        n210 = xnode ("Register Read")() -> ("Data"=w549:u64)  [unwired: 1 in, 1 out]
        n211 = xnode ("Register Read")() -> ("Data"=w550:u64)  [unwired: 1 in, 1 out]
        n212 = xnode ("Register Read")() -> ("Data"=w548:u64)  [unwired: 1 in, 1 out]
        n213 = Increment(x=w553) -> (x+1=w551:u64)
        n214 = xnode ("Register Write")("Data"=w551) -> ()  [unwired: 1 in, 1 out]
        n215 = Bundle By Name(cluster=w556, "State"=DisplacementStates."MoveErrorCode", "Sensor"=u8 1, "ErrorSample.RxFrames"=w551, "ErrorSample.TxBytes"=w550, "ErrorSample.RxBytes"=w549, "ErrorSample.TxFrames"=w548, "ErrorSample.Timestamp"=w547) -> (w555:T1)
      }
      frame "MoveErrorCode" {
        n216 = Unbundle By Name(w559) -> ("ErrorSample"=w557:T4)
        n217 = xnode ("FIFO Method Node")("Element"=w557, "Timeout"=0) -> ()  [unwired: 1 in, 2 out]
        n218 = Bundle By Name(cluster=w559, "State"=DisplacementStates."WaitForTrigger", "Sensor"=u8 1) -> (w562:T1)
      }
    }
  }
  n219 = node-c288(w2) -> ()
